vi "Self Update Example.vi"(8 "error in (no error)":errorcluster, 11 "SelfUpdate in":refnum<class "SelfUpdate.lvclass">) -> (0 "error out":errorcluster, 3 "SelfUpdate out":refnum<class "SelfUpdate.lvclass">)   [LabVIEW 2013, in "SelfUpdate.lvclass"]
uses:
  SelfUpdate.lvclass
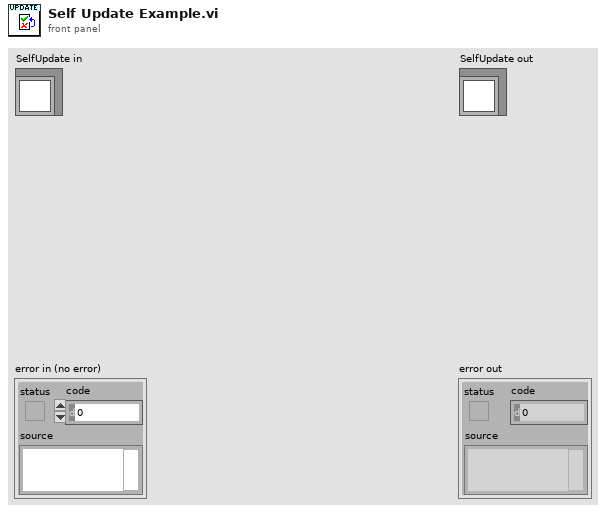
[diagram p1: front panel]
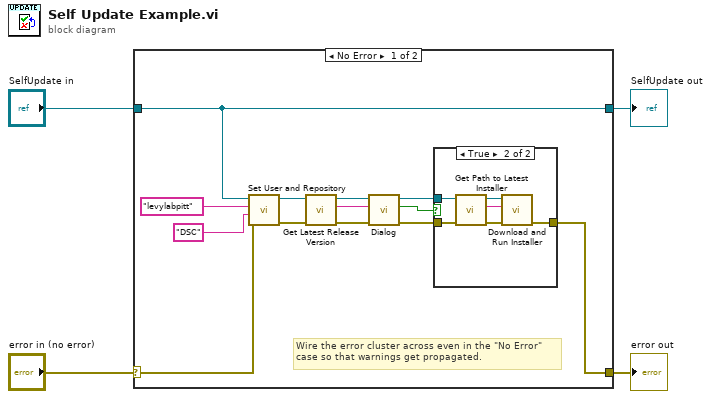
[diagram p0: block diagram]
diagram:
  n1 = case shown="No Error" "error in (no error)" {
    selector: "error in (no error)" -> [w12 w26]
    tunnel: [w11 w26] -> w3
    tunnel: [w17 w25] -> w1
    tunnel: "SelfUpdate in" -> [w17 w25]
    frame No Error {
      # "Wire the error cluster across even in the \"No Error\"\ncase so that warnings get propagated."
      n2 = call "Set User and Repository.vi"("error in (no error)"=w12, "Repository"="DSC" ("User"), "User"="levylabpitt", "SelfUpdate in"=w17) -> ("error out"=w15:errorcluster, "SelfUpdate out"=w16:refnum<class "SelfUpdate.lvclass">)  [unwired: 6 in]
      n3 = call "Get Latest Release Version.vi"("error in (no error)"=w15, "SelfUpdate in"=w16) -> ("error out"=w9:errorcluster, "latest tag"=w5:string, "SelfUpdate out"=w6:refnum<class "SelfUpdate.lvclass">)  [unwired: 7 in]
      n4 = call "Dialog.vi"("error in (no error)"=w9, "latest tag"=w5, "SelfUpdate in"=w6) -> ("error out"=w8:errorcluster, "T button?"=w10:bool, "SelfUpdate out"=w7:refnum<class "SelfUpdate.lvclass">)  [unwired: 6 in]
      n5 = case shown="True" w10 {
        tunnel: w8 -> [w18 w21]
        tunnel: w7 -> [_ w20]
        tunnel: [w18 w19] -> w11
        frame False {
        }
        frame True {
          n6 = call "Get Path to Latest Installer.vi"("error in (no error)"=w21, "SelfUpdate in"=w20) -> ("error out"=w22:errorcluster, "Path to download"=w24:string, "SelfUpdate out"=w23:refnum<class "SelfUpdate.lvclass">)  [unwired: 7 in]
          n7 = call "Download and Run Installer.vi"("error in (no error)"=w22, "path to download"=w24, "SelfUpdate in"=w23) -> ("error out"=w19:errorcluster)  [unwired: 7 in, 1 out]
        }
      }
    }
    frame Error {
    }
  }
  "error out" <- w3
  "SelfUpdate out" <- w1
